vi "estadoToneBurst_FastSlow.vi"(8 "error in (no error)":errorcluster, 10 "Tm":i32=60) -> (0 "error out":errorcluster)   [LabVIEW 2019, in "Prueba31.lvclass"]
uses:
  Prueba31.lvclass
panel:
  out "Tm":i32=60
  out "seg":i32=60
  in  "terminar":bool
  out "estado":string
  # "Tiempo de la prueba"
  # "Segundos"
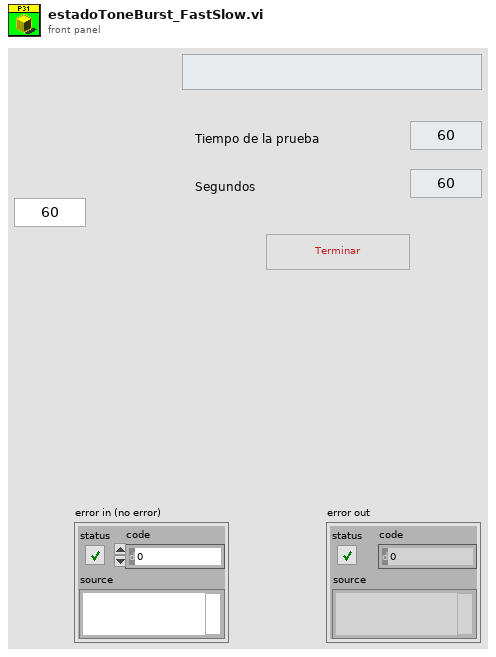
[diagram p1: front panel]
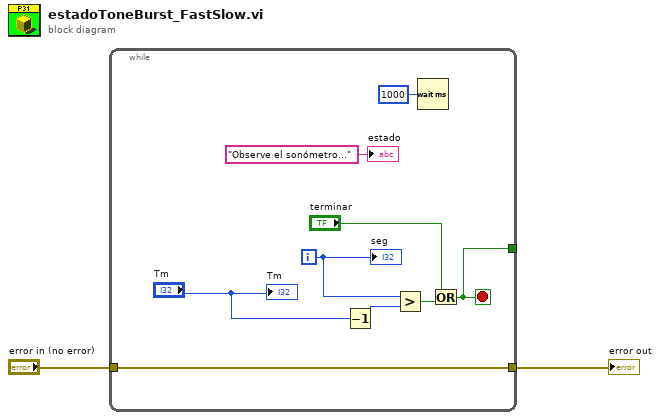
[diagram p0: block diagram]
diagram:
  n1 = while {
    tunnel: [w6] -> _
    tunnel: "error in (no error)" -> [w4]
    tunnel: [w4] -> w1
    i -> [w10]
    stop <- w6 stop-if-true
    n2 = Decrement(x="Tm") -> (x-1=w5:i32)
    n3 = Greater?(x=w10, y=w5) -> (0:w8:bool)
    n4 = Wait (ms)(milliseconds to wait=u32 1000) -> ()  [unwired: 1 out]
    n5 = Or(x="terminar", y=w8) -> (x .or. y?=w6:bool)
    "estado" <- "Observe el sonómetro..." ("estado")
    "seg" <- w10
    "Tm" <- "Tm"
  }
  "error out" <- w1
